vi "Run Master.vi"(11 "NXT/EV3 in":T1) -> (3 "EV3 out":T1)   [LabVIEW 2016]
uses:
  <vilib>/NXT/Subs/LVHSConnector.ctl
  <vilib>/NXT/LegoClasses/BrickReference/BrickReference.lvclass
  <vilib>/NXT/Block Support/NXT_ButtonSelector.ctl
  <vilib>/NXT/Dual Mode Library/Waits/Wait_Btn_Press.vi
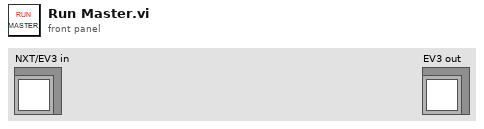
[diagram p1: front panel]
types:
  T1 = typedef "LVHSConnector.ctl" = refnum<class "BrickReference.lvclass">
  T2 = typedef "NXT_ButtonSelector.ctl" = u16
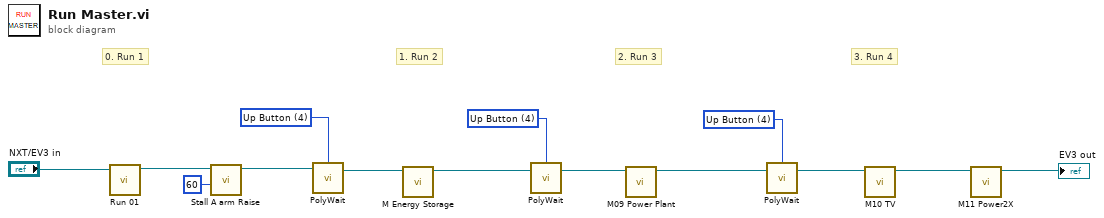
[diagram p0: block diagram]
diagram:
  w10 = T2 4 items=["Enter button"=3, "Left button"=2, "Right button"=1, "Up Button"=4, "Down Button"=5] ("Button (Enter button)")
  w11 = T2 4 items=["Enter button"=3, "Left button"=2, "Right button"=1, "Up Button"=4, "Down Button"=5] ("Button (Enter button)")
  w14 = T2 4 items=["Enter button"=3, "Left button"=2, "Right button"=1, "Up Button"=4, "Down Button"=5] ("Button (Enter button)")
  # "0. Run 1"
  # "3. Run 4"
  # "2. Run 3"
  # "1. Run 2"
  n1 = call "Run 01.vi"("NXT/EV3 in"="NXT/EV3 in") -> ("EV3 out"=w3:T1)  [unwired: 10 in]
  n2 = call "Stall A arm Raise.vi"("Power"=i8 60, "NXT/EV3"=w3) -> ("NXT/EV3"=w1:T1)  [unwired: 9 in]
  n3 = call-poly <vilib>:"PolyWait.vi"("NXT/EV3"=w1, "Button (Enter button)"=w14) -> ("NXT/EV3"=w13:T1)  [unwired: 2 in]
  n4 = call "M Energy Storage.vi"("NXT/EV3"=w13) -> ("EV3 out"=w7:T1)  [unwired: 10 in]
  n5 = call-poly <vilib>:"PolyWait.vi"("NXT/EV3"=w7, "Button (Enter button)"=w11) -> ("NXT/EV3"=w12:T1)  [unwired: 2 in]
  n6 = call "M09 Power Plant.vi"("EV3 in"=w12) -> ("EV3 out"=w9:T1)  [unwired: 10 in]
  n7 = call-poly <vilib>:"PolyWait.vi"("NXT/EV3"=w9, "Button (Enter button)"=w10) -> ("NXT/EV3"=w8:T1)  [unwired: 2 in]
  n8 = call "M10 TV.vi"("NXT/EV3"=w8) -> ("EV3 out"=w6:T1)  [unwired: 10 in]
  n9 = call "M11 Power2X.vi"("NXT/EV3"=w6) -> ("EV3 out"=→"EV3 out":T1)  [unwired: 10 in]
